vi "Stop Core.vi"(10 "final error code":i32, 11 "Actor Template in":refnum<class "Actor Template.lvclass">) -> (3 "Actor Template out":refnum<class "Actor Template.lvclass">)   [LabVIEW 2012, in "Actor Template.lvlib" / "Actor Template.lvclass"]
uses:
  Actor Template.lvclass
  <vilib>/ActorFramework/Actor/Actor.lvclass
  Actor Template.lvclass/Actor Template.ctl
  <vilib>/ActorFramework/Stop Msg/Stop Msg.lvclass/Stop Msg.ctl
  <vilib>/ActorFramework/Message Enqueuer/Message Enqueuer.lvclass/Message Enqueuer.ctl
  <vilib>/ActorFramework/Stop Msg/Send Emergency Stop.vi
  <vilib>/ActorFramework/Stop Msg/Send Normal Stop.vi
  <vilib>/ActorFramework/Message Enqueuer/Enqueue Critical.vi
  <vilib>/ActorFramework/Message Enqueuer/Enqueue.vi
  <vilib>/ActorFramework/Message Priority Queue/Priority Enqueue.vi
  <vilib>/ActorFramework/Stop Msg/Stop Msg.lvclass
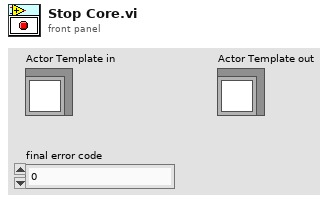
[diagram p1: front panel]
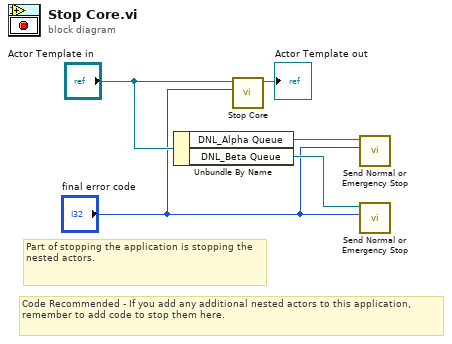
[diagram p0: block diagram]
diagram:
  # "Code Recommended - If you add any additional nested actors to this application, remember to add code to stop them here."
  # "Part of stopping the application is stopping the nested actors."
  n1 = Unbundle By Name("Actor Template in") -> ("DNL_Alpha Queue"=w3:refnum<class "Message Enqueuer.lvclass">, "DNL_Beta Queue"=w2:refnum<class "Message Enqueuer.lvclass">)
  n2 = call-parent "Stop Core.vi"("final error code"="final error code", "Actor in"="Actor Template in") -> ("Actor out"=→"Actor Template out":refnum<class "Actor Template.lvclass">)  [unwired: 9 in]
  n3 = call <vilib>:"Send Normal or Emergency Stop.vi"("final error code"="final error code", "Message Enqueuer"=w3) -> ()  [unwired: 9 in, 1 out]
  n4 = call <vilib>:"Send Normal or Emergency Stop.vi"("final error code"="final error code", "Message Enqueuer"=w2) -> ()  [unwired: 9 in, 1 out]
